vi "GetServerError.vi"(8 "ROS":T1={"topic port"=1236, "Node"="/labview", "topic"="/robot/head/command_head_nod", "type"="std_msgs/Bool", "node port"=7000, "error "={"status"=FALSE, "code"=0, "source"=""}, "Direction"=enum."Publisher", "APIs"=[], "Update (ms)"=1, "write queue"=1}, 9 "Err in":string, 10 "Cmd log":T3[](array[typedef]), 11 "error log path":path) -> ()   [LabVIEW 2012]
uses:
  <userlib>/ROSforLV/ROS/Code/Console/Servers/ServerSubs/ROSLog.ctl
  <userlib>/ROSforLV/ROS/Code/SubVIs/_ROSControl.ctl
  <userlib>/ROSforLV/ROS/Code/SubVIs/_ROSDirection.ctl
panel:
  out "subarray":T3[](array[typedef])
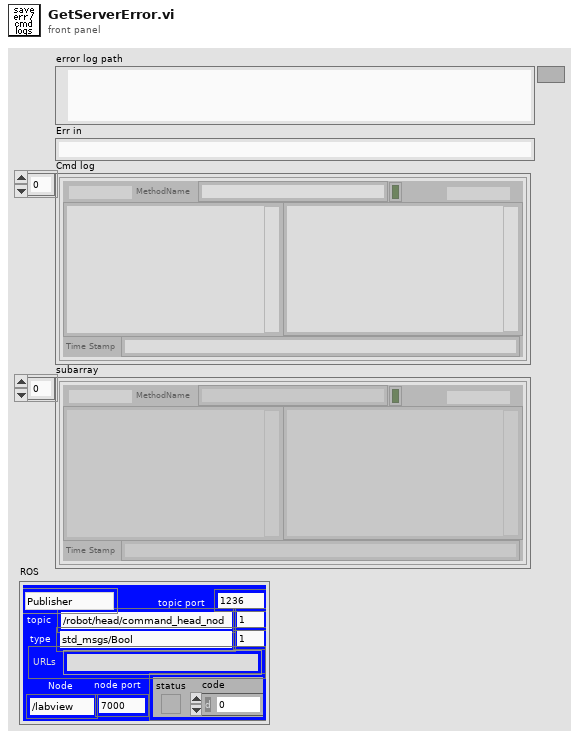
[diagram p1: front panel]
types:
  T1 = typedef "_ROSControl.ctl" = cluster{"topic port":u16, "Node":string, "topic":string, "type":string, "node port":u32, "error ":errorcluster, "Direction":T2, "APIs":string[], "Update (ms)":u16, "write queue":u16}
  T2 = typedef "_ROSDirection.ctl" = enum16{"Node", "Publisher", "Subscriber", "Service Client"}
  T3 = typedef "ROSLog.ctl" = cluster{"Sent":string, "Reply":string, "MethodName":string, "success":bool, "Dir1":string, "Dir2":string, "Time Stamp":string}
  T4 = cluster{"[0]":T3, "[1]":T3, "[2]":T3, "[3]":T3, "[4]":T3, "[5]":T3, "[6]":T3, "[7]":T3, "[8]":T3}
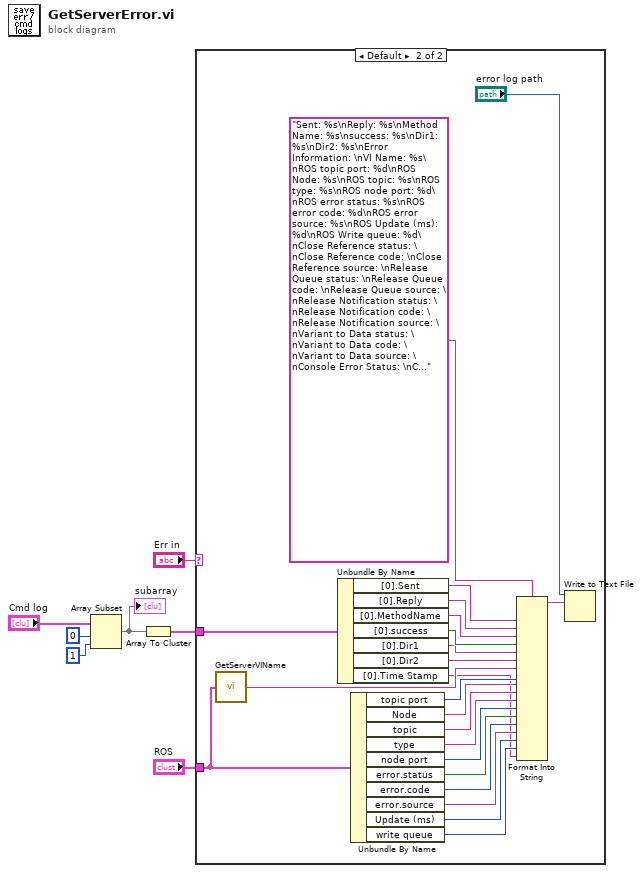
[diagram p0: block diagram]
diagram:
  n1 = Array Subset(array="Cmd log", index=0, length=1) -> (w3:T3[])
  "subarray" <- w3
  n2 = Array To Cluster(array=w3) -> (cluster=w1:T4)
  n3 = case shown="Default" "Err in" {
    tunnel: "ROS" -> [_ w20]
    tunnel: w1 -> [_ w21]
    frame "" {
    }
    frame Default {
      n4 = call <userlib>:"GetServerVIName.vi"("ROS"=w20) -> ("vi name"=w19:string)
      n5 = Unbundle By Name(w21) -> ("[0].Sent"=w27:string, "[0].Reply"=w26:string, "[0].MethodName"=w25:string, "[0].success"=w24:bool, "[0].Dir1"=w23:string, "[0].Dir2"=w22:string, "[0].Time Stamp"=w8:string)
      n6 = Unbundle By Name(w20) -> ("topic port"=w18:u16, "Node"=w17:string, "topic"=w16:string, "type"=w15:string, "node port"=w14:u32, "error.status"=w13:bool, "error.code"=w12:i32, "error.source"=w11:string, "Update (ms)"=w10:u16, "write queue"=w9:u16)
      n7 = Format Into String(format string="Sent: %s\nReply: %s\nMethod Name: %s\nsuccess: %s\nDir1: %s\nDir2: %s\nError Information: \nVI Name: %s\nROS topic port: %d\nROS Node: %s\nROS topic: %s\nROS type: %s\nROS node port: %d\nROS error status: %s\nROS error code: %d\nROS error source: %s\nROS Update (ms): %d\nROS Write queue: %d\nClose Reference status: \nClose Reference code: \nClose Reference source: \nRelease Queue status: \nRelease Queue code: \nRelease Queue source: \nRelease Notification status: \nRelease Notification code: \nRelease Notification source: \nVariant to Data status: \nVariant to Data code: \nVariant to Data source: \nConsole Error Status: \nConsole Error Code: \nConsole Error Source: \nTimestamp: %s", w27, w26, w25, w24, w23, w22, w19, w18, w17, w16, w15, w14, w13, w12, w11, w10, w9, w8) -> (resulting string=w29:string)  [unwired: 2 in, 1 out]
      n8 = Write to Text File(file (use dialog)="error log path", text=w29) -> ()  [unwired: 2 in, 3 out]
    }
  }
